vi "Unpowered Analog Output Data.vi"(8 "error in (no error)":errorcluster, 10 "Unpowered Analog Output (3:3)":u16(ring)=3 items=["3"=3, "4"=4], 11 "VISA resource name":refnum<visa-resource-name>) -> (0 "error out":errorcluster, 2 "Output Value":dbl format="%.1f", 3 "VISA resource name out":refnum<visa-resource-name>)   [LabVIEW 2012, in "Lake Shore 336.lvlib"]
doc: "This VI returns the Unpowered Output value. This is for the unpowered analog outputs 3 and 4 only. Use the Heater Output Data.VI for outputs 1 and 2."
uses:
  Lake Shore 336.lvlib
  Instance           1 36Saved   Unpowered Analog Output Data .vi
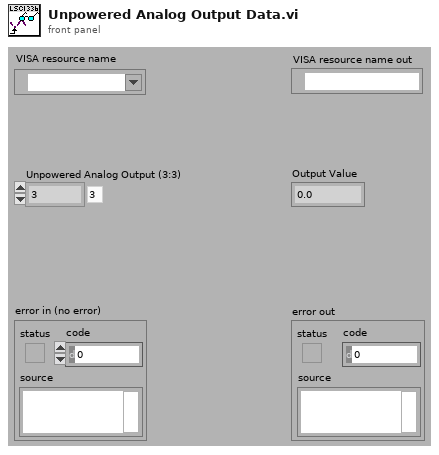
[diagram p1: front panel]
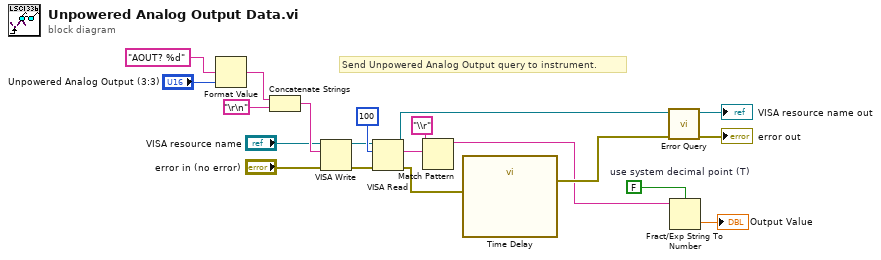
[diagram p0: block diagram]
diagram:
  w6 = FALSE  # use system decimal point (T)
  # "Send Unpowered Analog Output query to instrument."
  n1 = Format Value(format string="AOUT? %d", value (0)="Unpowered Analog Output (3:3)") -> (output string=w1:string)  [unwired: 1 in]
  n2 = Concatenate Strings(w1, "\r\n") -> (w11:string)
  n3 = VISA Write(VISA resource name="VISA resource name", write buffer=w11, error in (no error)="error in (no error)") -> (VISA resource name out=w15:refnum<visa-resource-name>, error out=w14:errorcluster)  [unwired: 1 out]
  n4 = VISA Read(VISA resource name=w15, byte count=100, error in (no error)=w14) -> (VISA resource name out=w9:refnum<visa-resource-name>, read buffer=w17:string, error out=w13:errorcluster)  [unwired: 1 out]
  n5 = Match Pattern(string=w17, regular expression="\\r") -> (before substring=w5:string)  [unwired: 1 in, 3 out]
  n6 = call "Time Delay"("error in (no error)"=w13) -> ("error out"=w10:errorcluster)  [unwired: 10 in]
  n7 = call "Error Query.vi"("error in (no error)"=w10, "VISA resource name"=w9) -> ("error out"=→"error out":errorcluster, "VISA resource name out"=→"VISA resource name out":refnum<visa-resource-name>)  [unwired: 7 in, 1 out]
  n8 = Fract/Exp String To Number(use system decimal point (T)=w6, string=w5) -> (number=→"Output Value":dbl)  [unwired: 2 in, 1 out]
